vi "Exit Test Bench.vi"(5 "timeout ms (-1)":i32=-1, 8 "error in (no error)":errorcluster, 11 "Info":string) -> (0 "error out":errorcluster)   [LabVIEW 2019, in "Test Bench Tools.lvlib"]
uses:
  Test Bench Tools.lvlib
  TB Global 1.vi
  <resource>/objmgr/ni.dex.rc
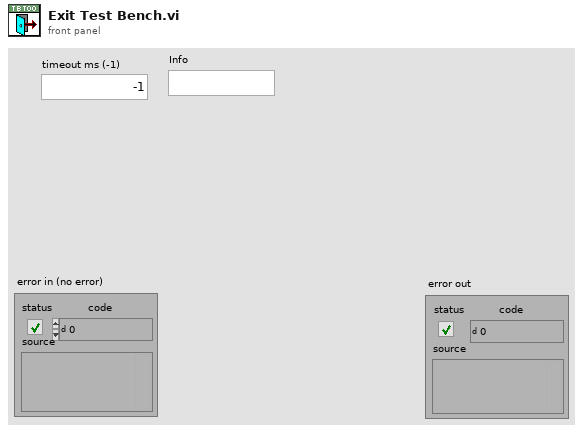
[diagram p1: front panel]
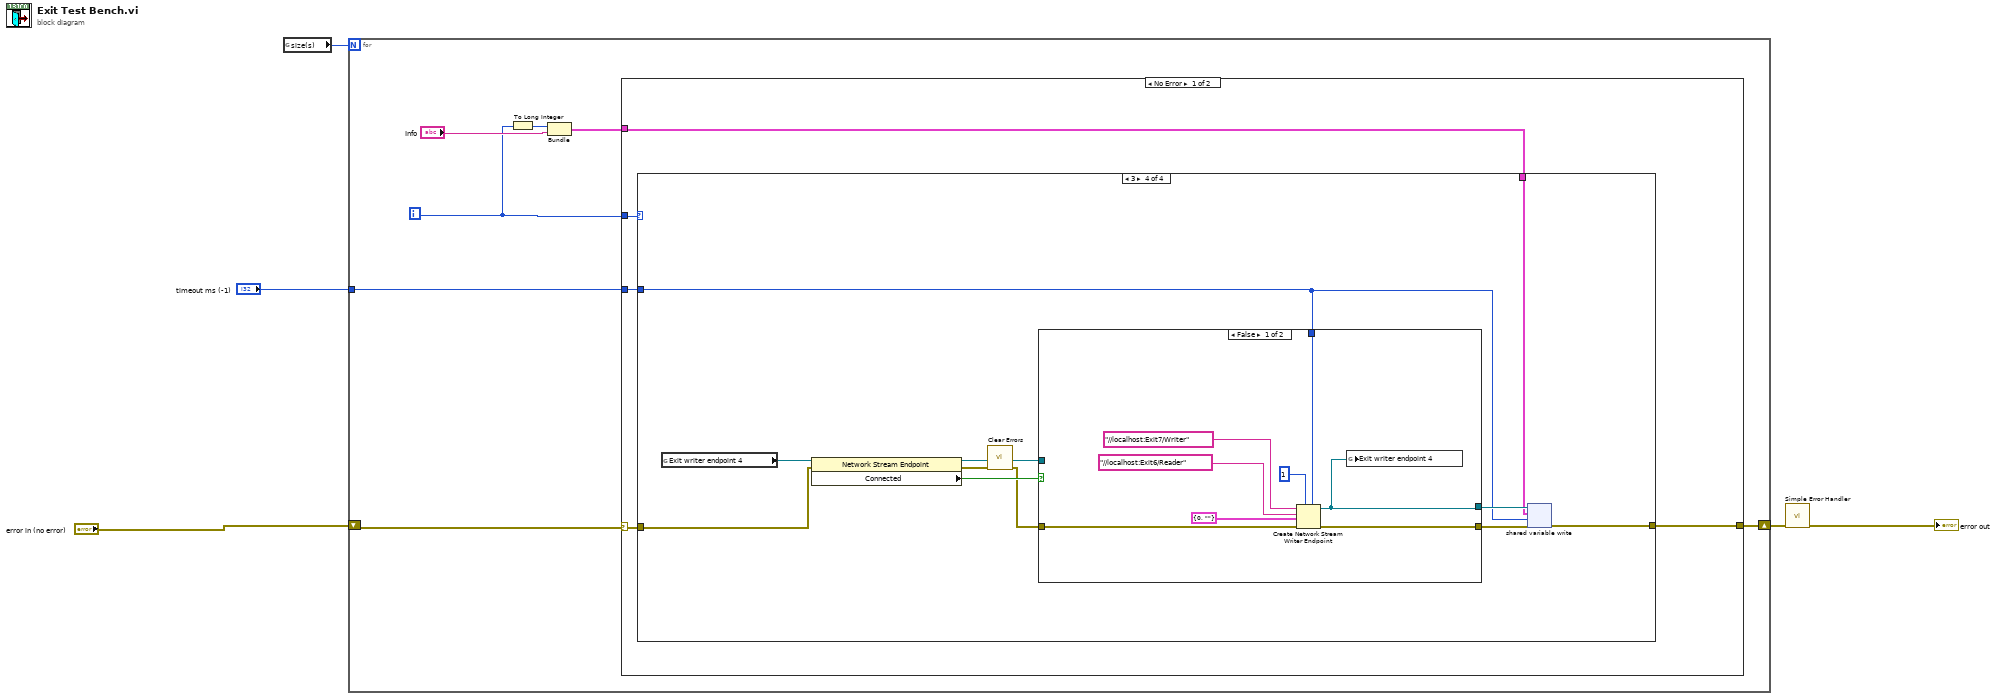
[diagram p0: block diagram]
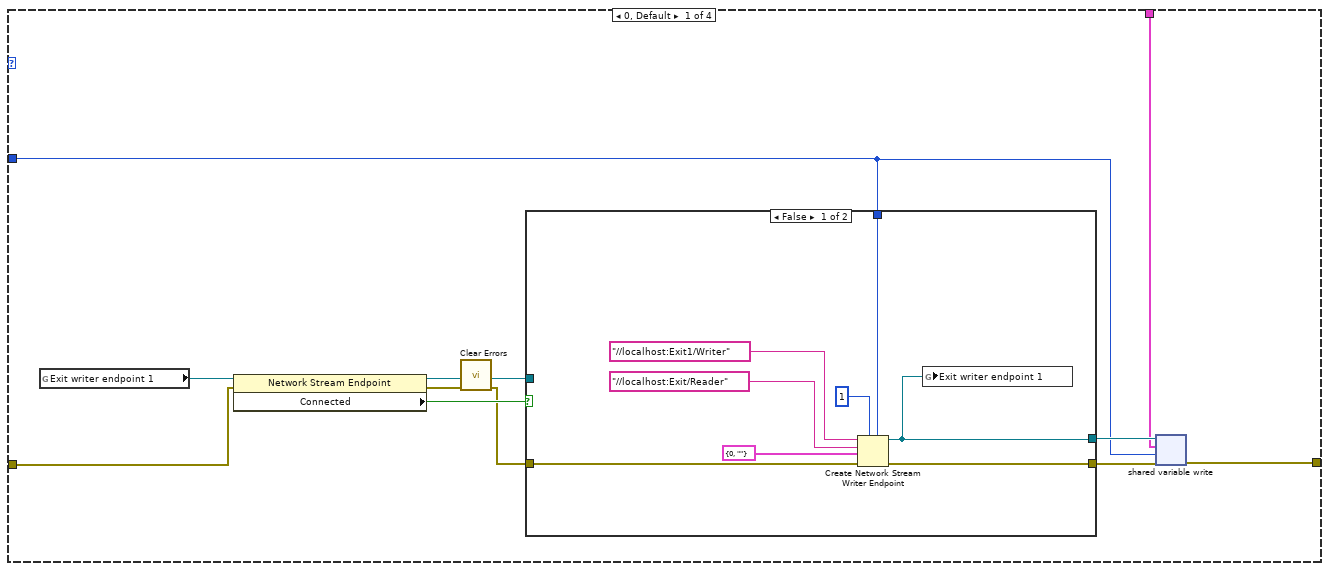
[diagram p2: hidden frame]
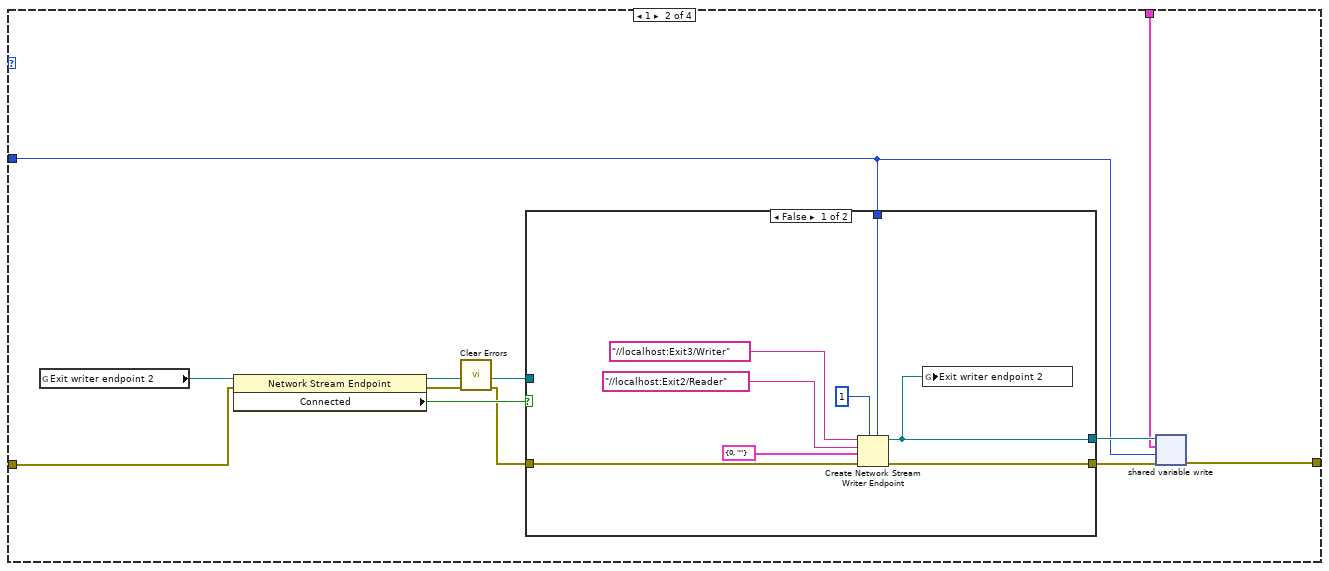
[diagram p4: hidden frame]
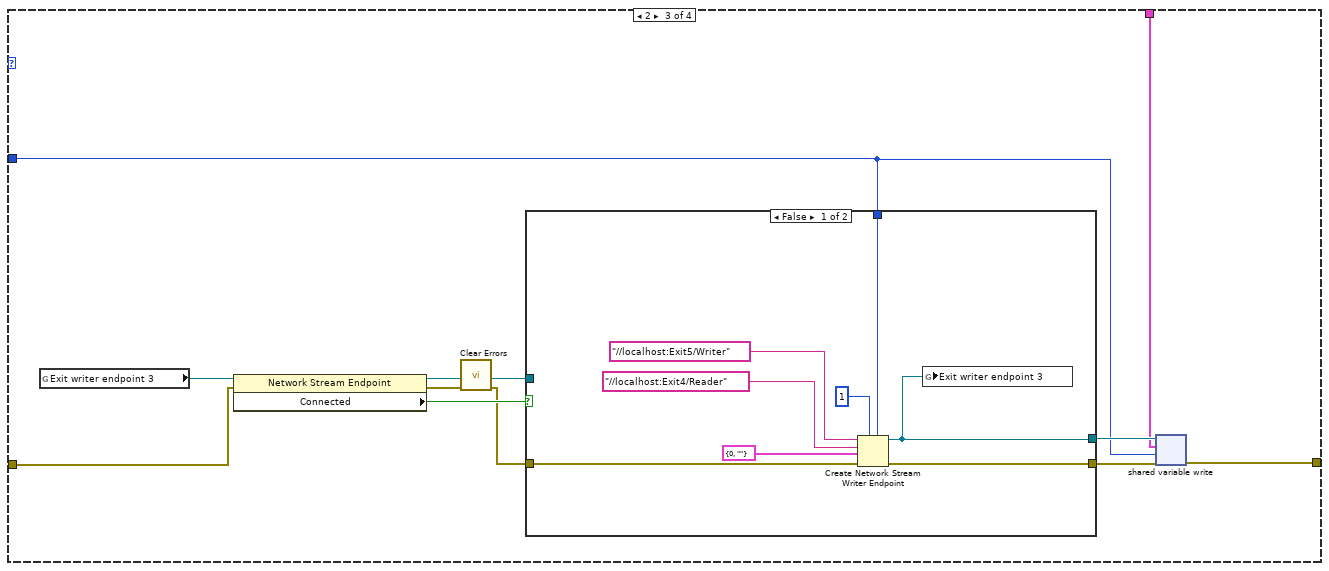
[diagram p6: hidden frame]
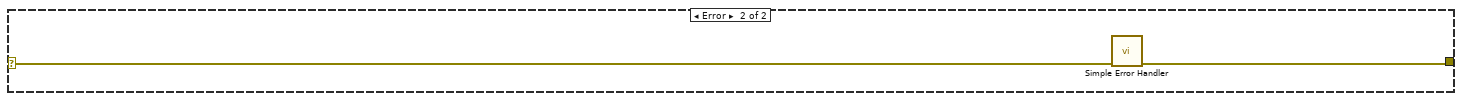
[diagram p9: hidden frame]
diagram:
  n1 = global read "TB Global 1.vi" "size(s)"() -> (w2:i32)
  n2 = for {
    N: w2 -> [_]
    shift-right: [w11] -> w5
    shift-left: "error in (no error)" -> [w10]
    tunnel: "timeout ms (-1)" -> [w6]
    i -> [w7]
    n3 = To Long Integer(number=w7) -> (32bit integer=w8:i32)
    n4 = Bundle(w8, "Info"="Info") -> (w12:cluster{i32, "Info":string})  [unwired: 1 in]
    n5 = case shown="No Error" w10 {
      selector: w10 -> [w16 w103]
      tunnel: w6 -> [w15 _]
      tunnel: w12 -> [w14 _]
      tunnel: [w17 w102] -> w11
      tunnel: w7 -> [w13 _]
      frame No Error {
        n6 = case shown="3" w13 {
          tunnel: [w22 w43 w64 w85] -> w17
          tunnel: w16 -> [w21 w42 w63 w84]
          tunnel: w15 -> [w19 w40 w61 w82]
          tunnel: w14 -> [w18 w39 w60 w81]
          frame 0, Default {
            n7 = global read "TB Global 1.vi" "Exit writer endpoint 1"() -> (w26:refnum<k21>)
            n8 = property class="Network Stream Endpoint"(reference=w26, error in=w21) -> (reference out=w23:refnum<k21>, error out=w25:errorcluster, "Connected"=w24:bool)
            n9 = call <vilib>:"Clear Errors.vi"("error in (no error)"=w25) -> ("error out"=w20:errorcluster)  [unwired: 5 in, 1 out]
            n10 = case shown="False" w24 {
              tunnel: [w29 w38] -> w28
              tunnel: [w30 w37] -> w27
              tunnel: w20 -> [w32 w37]
              tunnel: w23 -> [_ w38]
              tunnel: w19 -> [w31 _]
              frame False {
                n11 = Create Network Stream Writer Endpoint(5:w31, 7:1 ("writer buffer size"), 8:w32, 9:cluster{"Socket":i32, "Info":string} {"Socket"=0, "Info"=""}, 10:"//localhost:Exit/Reader" ("reader name"), 11:"//localhost:Exit1/Writer" ("reader name")) -> (0:w30:errorcluster, 3:w29:refnum<k21>)  [unwired: 1 in]
                n12 = global write "TB Global 1.vi" "Exit writer endpoint 1"(w29) -> ()
              }
              frame True {
              }
            }
            n13 = shared-variable-write(w28, w27, w18, w19) -> (w22:errorcluster)  [unwired: 2 out]
          }
          frame 1 {
            n14 = global read "TB Global 1.vi" "Exit writer endpoint 2"() -> (w47:refnum<k21>)
            n15 = property class="Network Stream Endpoint"(reference=w47, error in=w42) -> (reference out=w44:refnum<k21>, error out=w46:errorcluster, "Connected"=w45:bool)
            n16 = call <vilib>:"Clear Errors.vi"("error in (no error)"=w46) -> ("error out"=w41:errorcluster)  [unwired: 5 in, 1 out]
            n17 = case shown="False" w45 {
              tunnel: [w50 w59] -> w49
              tunnel: [w51 w58] -> w48
              tunnel: w41 -> [w53 w58]
              tunnel: w44 -> [_ w59]
              tunnel: w40 -> [w52 _]
              frame False {
                n18 = Create Network Stream Writer Endpoint(5:w52, 7:1 ("writer buffer size"), 8:w53, 9:cluster{"Socket":i32, "Info":string} {"Socket"=0, "Info"=""}, 10:"//localhost:Exit2/Reader" ("reader name"), 11:"//localhost:Exit3/Writer" ("reader name")) -> (0:w51:errorcluster, 3:w50:refnum<k21>)  [unwired: 1 in]
                n19 = global write "TB Global 1.vi" "Exit writer endpoint 2"(w50) -> ()
              }
              frame True {
              }
            }
            n20 = shared-variable-write(w49, w48, w39, w40) -> (w43:errorcluster)  [unwired: 2 out]
          }
          frame 2 {
            n21 = global read "TB Global 1.vi" "Exit writer endpoint 3"() -> (w68:refnum<k21>)
            n22 = property class="Network Stream Endpoint"(reference=w68, error in=w63) -> (reference out=w65:refnum<k21>, error out=w67:errorcluster, "Connected"=w66:bool)
            n23 = call <vilib>:"Clear Errors.vi"("error in (no error)"=w67) -> ("error out"=w62:errorcluster)  [unwired: 5 in, 1 out]
            n24 = case shown="False" w66 {
              tunnel: [w71 w80] -> w70
              tunnel: [w72 w79] -> w69
              tunnel: w62 -> [w74 w79]
              tunnel: w65 -> [_ w80]
              tunnel: w61 -> [w73 _]
              frame False {
                n25 = Create Network Stream Writer Endpoint(5:w73, 7:1 ("writer buffer size"), 8:w74, 9:cluster{"Socket":i32, "Info":string} {"Socket"=0, "Info"=""}, 10:"//localhost:Exit4/Reader" ("reader name"), 11:"//localhost:Exit5/Writer" ("reader name")) -> (0:w72:errorcluster, 3:w71:refnum<k21>)  [unwired: 1 in]
                n26 = global write "TB Global 1.vi" "Exit writer endpoint 3"(w71) -> ()
              }
              frame True {
              }
            }
            n27 = shared-variable-write(w70, w69, w60, w61) -> (w64:errorcluster)  [unwired: 2 out]
          }
          frame 3 {
            n28 = global read "TB Global 1.vi" "Exit writer endpoint 4"() -> (w89:refnum<k21>)
            n29 = property class="Network Stream Endpoint"(reference=w89, error in=w84) -> (reference out=w86:refnum<k21>, error out=w88:errorcluster, "Connected"=w87:bool)
            n30 = call <vilib>:"Clear Errors.vi"("error in (no error)"=w88) -> ("error out"=w83:errorcluster)  [unwired: 5 in, 1 out]
            n31 = case shown="False" w87 {
              tunnel: [w92 w101] -> w91
              tunnel: [w93 w100] -> w90
              tunnel: w83 -> [w95 w100]
              tunnel: w86 -> [_ w101]
              tunnel: w82 -> [w94 _]
              frame False {
                n32 = Create Network Stream Writer Endpoint(5:w94, 7:1 ("writer buffer size"), 8:w95, 9:cluster{"Socket":i32, "Info":string} {"Socket"=0, "Info"=""}, 10:"//localhost:Exit6/Reader" ("reader name"), 11:"//localhost:Exit7/Writer" ("reader name")) -> (0:w93:errorcluster, 3:w92:refnum<k21>)  [unwired: 1 in]
                n33 = global write "TB Global 1.vi" "Exit writer endpoint 4"(w92) -> ()
              }
              frame True {
              }
            }
            n34 = shared-variable-write(w91, w90, w81, w82) -> (w85:errorcluster)  [unwired: 2 out]
          }
        }
      }
      frame Error {
        n35 = call <vilib>:"Simple Error Handler.vi"("error in (no error)"=w103) -> ("error out"=w102:errorcluster)  [unwired: 4 in, 4 out]
      }
    }
  }
  n36 = call <vilib>:"Simple Error Handler.vi"("error in (no error)"=w5) -> ("error out"=→"error out":errorcluster)  [unwired: 4 in, 4 out]
